vi "Write Measurement Units.vi"(8 "error in":errorcluster, 10 "measurement units":T1, 11 "thermocouple channel in":refnum<class "Thermocouple Channel.lvclass">) -> (0 "error out":errorcluster, 3 "thermocouple channel out":refnum<class "Thermocouple Channel.lvclass">)   [LabVIEW 2017, in "Scan Engine Scripting.lvlib" / "Thermocouple Channel.lvclass"]
doc: "Writes the measurement units to the private data of the channel."
uses:
  Thermocouple Channel.lvclass
  Measurement Units.ctl
  Thermocouple Channel.lvclass/Thermocouple Channel.ctl
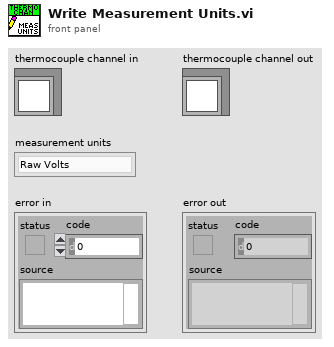
[diagram p1: front panel]
types:
  T1 = typedef "Scan Engine Scripting.lvlib/Thermocouple Channel.lvclass/Measurement Units.ctl" = enum16{"Raw Volts", "Degrees Kelvin", "Degrees Celsius", "Degrees Fahrenheit", "Degrees Rankine"}
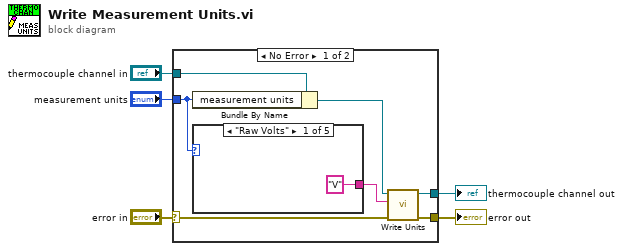
[diagram p0: block diagram]
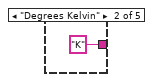
[diagram p2: hidden frame]
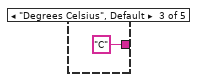
[diagram p3: hidden frame]
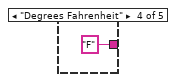
[diagram p4: hidden frame]
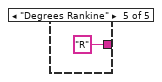
[diagram p5: hidden frame]
diagram:
  n1 = case shown="No Error" "error in" {
    selector: "error in" -> [w9 w18]
    tunnel: [w8 w18] -> w4
    tunnel: [w10 w19] -> w2
    tunnel: "thermocouple channel in" -> [w12 w19]
    tunnel: "measurement units" -> [w7 _]
    frame No Error {
      n2 = Bundle By Name(cluster=w12, "measurement units"=w7) -> (w11:refnum<class "Thermocouple Channel.lvclass">)
      n3 = case shown="\"Raw Volts\"" w7 {
        tunnel: ["V" "K" "C" "F" "R"] -> w6
        frame "Raw Volts" {
        }
        frame "Degrees Kelvin" {
        }
        frame "Degrees Celsius", Default {
        }
        frame "Degrees Fahrenheit" {
        }
        frame "Degrees Rankine" {
        }
      }
      n4 = call-dynamic "Write Units.vi"("error in"=w9, "units"=w6, "channel in"=w11) -> ("error out"=w8:errorcluster, "channel out"=w10:refnum<class "Thermocouple Channel.lvclass">)  [unwired: 7 in]
    }
    frame Error {
    }
  }
  "error out" <- w4
  "thermocouple channel out" <- w2
